vi "NMR_Long_RF_Pulse_Sequence_V4.vi"() -> ()   [LabVIEW 2020]
uses:
  <instrlib>/niFgen/niFgen.llb/niFgen Output Mode.ctl
  <instrlib>/niFgen/niFgen.llb/niFgen Waveform Type.ctl
  <instrlib>/niFgen/niFgen.llb/niFgen_ctl Trigger DigEdge - Edge Values (Ring).ctl
  <instrlib>/niFgen/niFgen.llb/niFgen_ctl Trigger Source Values (Ring).ctl
  <instrlib>/niFgen/niFgen.llb/niFgen Trigger Mode.ctl
  <instrlib>/niScope/Controls/niScope acquisition type.ctl
  <instrlib>/niScope/Controls/niScope trigger slope.ctl
  <instrlib>/niScope/Controls/niScope trigger source.ctl
  <vilib>/Analysis/2dsp.llb/Integral Method.ctl
  <vilib>/Analysis/8numeric.llb/1D Numeric Integration.vi
  <vilib>/Utility/file.llb/Read Delimited Spreadsheet (DBL).vi
  <instrlib>/niFgen/niFgen.llb/niFgen Create Waveform (DBL).vi
  <instrlib>/niScope/Configure/Trigger/niScope Configure Trigger Edge.vi
  <instrlib>/niFgen/niFgen.llb/niFgen Configure Digital Edge Start Trigger.vi
  <instrlib>/niScope/Acquire/Fetch/niScope Fetch Cluster.vi
  <vilib>/Waveform/WDTFileIO.llb/Export Waveform To Spreadsheet File.vi
  <vilib>/Analysis/NI_AALPro.lvlib
panel:
  out "Averaged T2 Decay":waveform(dbl)(graph)={"t0"=timestamp(0 s since 1904-01-01), "dt"=0.0025142857142857146, "Y"=array[865 elements]} caption="Waveform Graph"
  out "Pulse Echos - Current Scan":T1(graph) caption="Waveform Graph"
  in  "Write Output to File?":bool
  out "Scan Number":i32=1
  out "Signal Intensity (Integral)":dbl=0.2866310909595196 format="%0.4f"
  out "Extracted T2 Decay - Current Scan":waveform(dbl)(graph)={"t0"=timestamp(0 s since 1904-01-01), "dt"=0.0025142857142857146, "Y"=array[865 elements]} caption="Waveform Graph"
  in  "Pulse Train File":path=path "D:/Pulse Train - 4s Duration, 3170 Pulses, 1.25ms Tau.txt"
  in  "Larmor Frequency":dbl=27450000.0 caption="Frequency" format="%.4p"
  in  "Number of Scans":i32=16
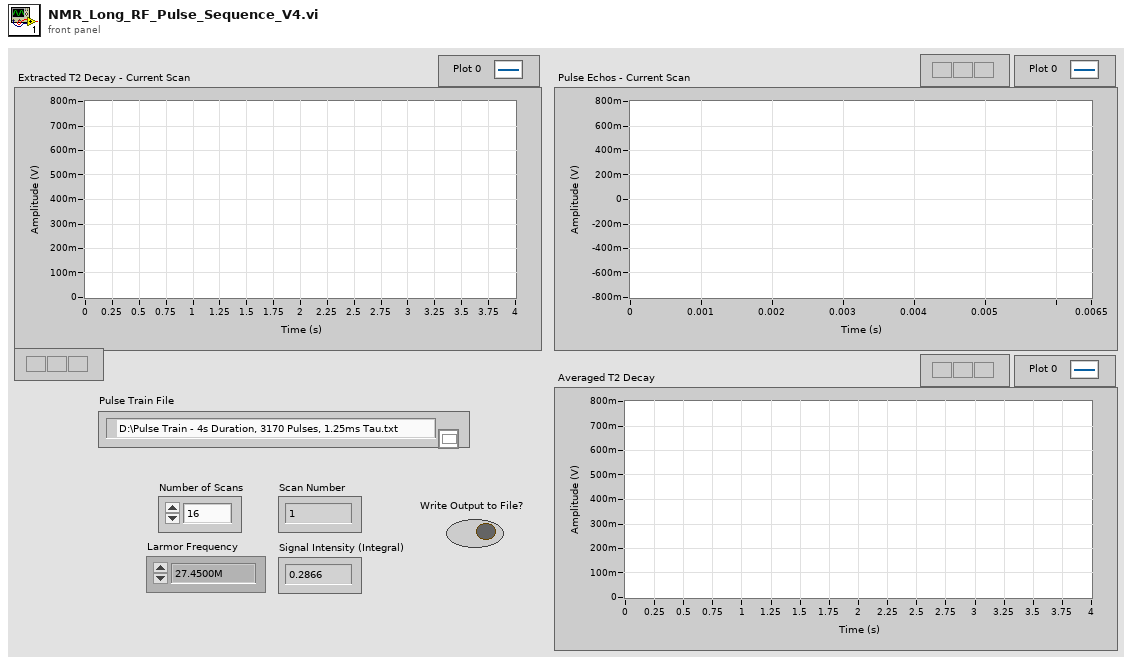
[diagram p1: front panel]
types:
  T1 = cluster{"relativeInitialX":dbl, "xIncrement":dbl, "wfm":dbl[]}
  T2 = typedef "niFgen Output Mode.ctl" = u32
  T3 = typedef "niScope trigger source.ctl" = string
  T4 = typedef "niFgen_ctl Trigger Source Values (Ring).ctl" = string
  T5 = typedef "NI_AALPro.lvlib/Integral Method.ctl" = i32
  T6 = typedef "niScope trigger slope.ctl" = i32
  T7 = typedef "niScope acquisition type.ctl" = i32
  T8 = typedef "niFgen Trigger Mode.ctl" = i32
  T9 = typedef "niFgen_ctl Trigger DigEdge - Edge Values (Ring).ctl" = i32
  T10 = typedef "niFgen Waveform Type.ctl" = i32
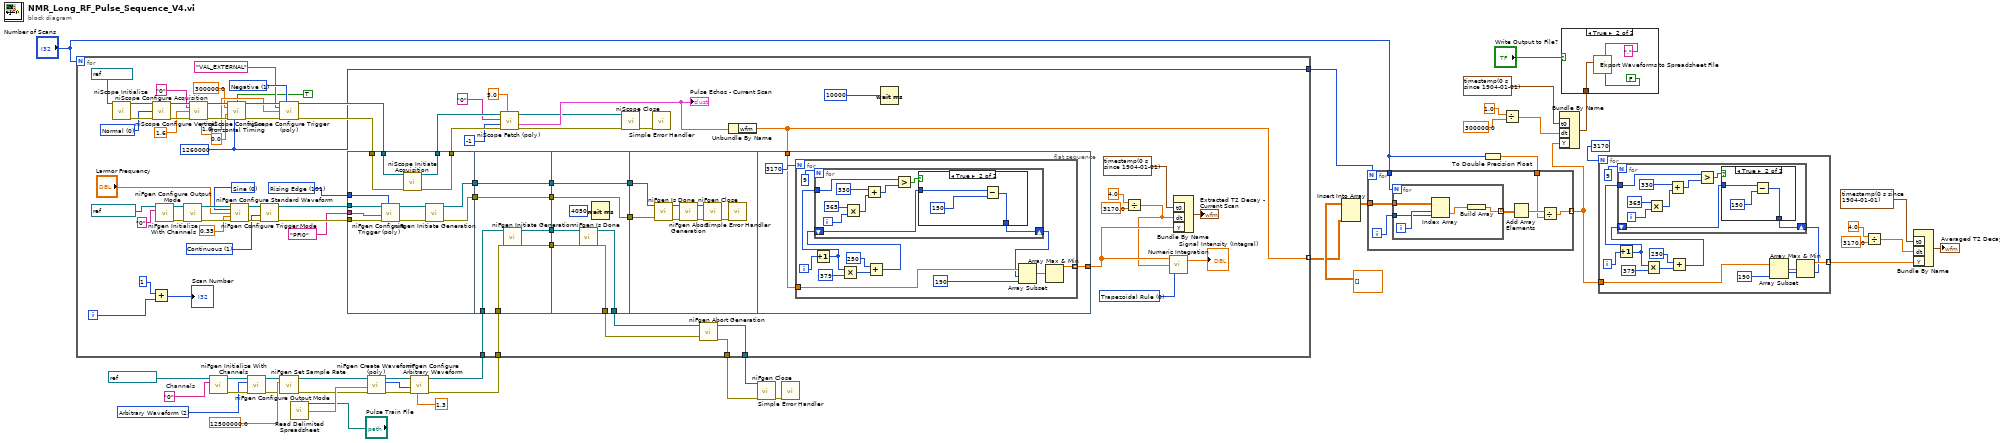
[diagram p0: block diagram]
diagram:
  w27 = "0"  # Channels
  w26 = T2 2 items=["Standard Function", "Frequency List", "Arbitrary Waveform", "Arbitrary Sequence", "Script"] ("output mode")
  n1 = call <instrlib>:"niFgen Initialize With Channels.vi"("Channel Name"=w27, "Resource Name"=refnum<k15> "PulseTrain" ("FGEN Resource Name 2")) -> ("error out"=w30:errorcluster, "Instrument Handle Out"=w31:refnum<k15>)  [unwired: 8 in]
  n2 = call <instrlib>:"niFgen Configure Output Mode.vi"("error in (no error)"=w30, "Output Mode (default: 0=Standard Function)"=w26, "Instrument Handle"=w31) -> ("error out"=w34:errorcluster, "Instrument Handle Out"=w33:refnum<k15>)  [unwired: 6 in]
  n3 = call <instrlib>:"niFgen Set Sample Rate.vi"("error in (no error)"=w34, "Sample Rate (Samp/s)"=12500000.0 ("Sample Rate"), "Instrument Handle"=w33) -> ("error out"=w37:errorcluster, "Instrument Handle Out"=w36:refnum<k15>)  [unwired: 7 in]
  n4 = call-poly <vilib>:"Read Delimited Spreadsheet.vi"("file path (dialog if empty)"="Pulse Train File") -> ("first row"=w38:dbl[])  [unwired: 9 in, 5 out]
  n5 = call-poly <instrlib>:"niFgen Create Waveform (poly).vi"("error in (no error)"=w37, "Waveform Data Array"=w38, "Instrument Handle"=w36) -> ("error out"=w40:errorcluster, "Waveform Handle"=w41:i32, "Instrument Handle Out"=w39:refnum<k15>)  [unwired: 6 in]
  n6 = call <instrlib>:"niFgen Configure Arbitrary Waveform.vi"("Gain"=1.3, "error in (no error)"=w40, "Waveform Handle"=w41, "Instrument Handle"=w39) -> ("error out"=w25:errorcluster, "Instrument Handle Out"=w24:refnum<k15>)  [unwired: 6 in]
  n7 = for {
    N: "Number of Scans" -> [_]
    tunnel: w25 -> [w96]
    tunnel: w24 -> [w95]
    tunnel: [w94] -> w22
    tunnel: [w93] -> w21
    tunnel: [w47] -> w18 mode=indexing
    tunnel: [w42] -> w9
    i -> [w50]
    w52 = T5 0 items=["Trapezoidal Rule", "Simpson's Rule", "Simpson's 3/8 Rule", "Bode Rule"] ("integration method")
    w42 = 1260000 ("min record length")
    w81 = T6 1 items=["Positive", "Negative"] ("trigger slope")
    w82 = T7 0 items=["Normal"=0, "Flex Res"=1, "DDC"=3] ("acquisition Type")
    w101 = T8 1 items=["Single", "Continuous", "Stepped", "Burst"] ("Trigger Mode (default: 1=continuous)")
    w105 = T9 101 items=["Rising Edge"=101, "Falling Edge"=102] ("Edge (Rising)")
    w106 = T10 0 items=["Sine", "Square", "Triangle", "Ramp Up", "Ramp Down", "DC", "Noise", "User"] ("Waveform")
    n8 = call <instrlib>:"niScope Initialize.vi"("resource name"=refnum<k15> "OScope") -> ("instrument handle"=w83:refnum<k15>, "error out"=w84:errorcluster)  [unwired: 13 in]
    n9 = call <instrlib>:"niScope Configure Acquisition.vi"("instrument handle"=w83, "acquisition Type"=w82, "error in"=w84) -> ("instrument handle out"=w86:refnum<k15>, "error out"=w87:errorcluster)  [unwired: 11 in]
    n10 = Add(x=1, y=w50) -> (x+y=→"Scan Number":i32)
    n11 = call <instrlib>:"niFgen Initialize With Channels.vi"("Channel Name"="0", "Resource Name"=refnum<k15> "FuncGen" ("Sine Wave Module")) -> ("error out"=w111:errorcluster, "Instrument Handle Out"=w114:refnum<k15>)  [unwired: 8 in]
    n12 = call <instrlib>:"niFgen Configure Output Mode.vi"("error in (no error)"=w111, "Instrument Handle"=w114) -> ("error out"=w110:errorcluster, "Instrument Handle Out"=w113:refnum<k15>)  [unwired: 7 in]
    n13 = call <instrlib>:"niScope Configure Vertical.vi"("instrument handle"=w86, "channels"="0", "vertical range"=1.6, "error in"=w87) -> ("instrument handle out"=w88:refnum<k15>, "error out"=w89:errorcluster)  [unwired: 10 in]
    n14 = call <instrlib>:"niScope Configure Horizontal Timing.vi"("instrument handle"=w88, "enforce realtime"=TRUE, "min sample rate"=300000.0, "reference position"=0.0, "error in"=w89, "min record length"=w42) -> ("instrument handle out"=w90:refnum<k15>, "error out"=w91:errorcluster)  [unwired: 8 in]
    n15 = call <instrlib>:"niFgen Configure Standard Waveform.vi"("Instrument Handle"=w113, "Waveform"=w106, "Frequency"="Larmor Frequency", "Amplitude"=0.35, "error in (no error)"=w110) -> ("Instrument Handle Out"=w112:refnum<k15>, "error out"=w109:errorcluster)  [unwired: 9 in]
    n16 = call <instrlib>:"niFgen Configure Trigger Mode.vi"("error in (no error)"=w109, "Trigger Mode (default: 1=continuous)"=w101, "Instrument Handle"=w112) -> ("error out"=w104:errorcluster, "Instrument Handle Out"=w102:refnum<k15>)  [unwired: 7 in]
    n17 = call-poly <instrlib>:"niScope Configure Trigger (poly).vi"("instrument handle"=w90, "trigger slope"=w81, "trigger source"=T3 "VAL_EXTERNAL", "trigger level"=1.0, "error in"=w91) -> ("instrument handle out"=w75:refnum<k15>, "error out"=w74:errorcluster)  [unwired: 9 in]
    n18 = flat-sequence {
      tunnel: w105 -> [w125]
      tunnel: w104 -> [w124]
      tunnel: T4 "PFI0" ("Source") -> [w123]
      tunnel: w102 -> [w122]
      tunnel: w75 -> [w120]
      tunnel: w74 -> [w119]
      tunnel: [w118] -> w73
      tunnel: [w117] -> w72
      tunnel: [w116] -> w62
      tunnel: [w115] -> w59
      tunnel: w96 -> [w132]
      tunnel: w95 -> [w131]
      tunnel: [w130] -> w66
      tunnel: [w129] -> w65
      tunnel: [w128] -> w63
      tunnel: w62 -> [w128]
      tunnel: [w127] -> w60
      tunnel: w59 -> [w127]
      tunnel: [w138] -> w99
      tunnel: [w137] -> w98
      tunnel: w66 -> [w136]
      tunnel: w65 -> [w135]
      tunnel: [w134] -> w64
      tunnel: w63 -> [w134]
      tunnel: [w133] -> w61
      tunnel: w60 -> [w133]
      tunnel: w64 -> [w141]
      tunnel: w61 -> [w140]
      tunnel: w47 -> [w148]
      tunnel: [w147] -> w54
      frame #0 {
        n19 = call-poly <instrlib>:"niFgen Configure Trigger (poly).vi"("Edge (Rising)"=w125, "error in (no error)"=w124, "Source"=w123, "Instrument Handle"=w122) -> ("error out"=w121:errorcluster, "Instrument Handle Out"=w126:refnum<k15>)  [unwired: 6 in]
        n20 = call <instrlib>:"niScope Initiate Acquisition.vi"("instrument handle"=w120, "error in"=w119) -> ("instrument handle out"=w118:refnum<k15>, "error out"=w117:errorcluster)  [unwired: 12 in]
        n21 = call <instrlib>:"niFgen Initiate Generation.vi"("error in (no error)"=w121, "Instrument Handle"=w126) -> ("error out"=w115:errorcluster, "Instrument Handle Out"=w116:refnum<k15>)  [unwired: 8 in]
      }
      frame #1 {
        n22 = call <instrlib>:"niFgen Initiate Generation.vi"("error in (no error)"=w132, "Instrument Handle"=w131) -> ("error out"=w129:errorcluster, "Instrument Handle Out"=w130:refnum<k15>)  [unwired: 8 in]
      }
      frame #2 {
        n23 = call <instrlib>:"niFgen Is Done.vi"("error in (no error)"=w135, "Instrument Handle"=w136) -> ("error out"=w138:errorcluster, "Instrument Handle Out"=w137:refnum<k15>)  [unwired: 7 in, 1 out]
        n24 = Wait (ms)(milliseconds to wait=u32 4050) -> ()  [unwired: 1 out]
      }
      frame #3 {
        n25 = call <instrlib>:"niFgen Is Done.vi"("error in (no error)"=w140, "Instrument Handle"=w141) -> ("error out"=w144:errorcluster, "Instrument Handle Out"=w143:refnum<k15>)  [unwired: 7 in, 1 out]
        n26 = call <instrlib>:"niFgen Abort Generation.vi"("error in (no error)"=w144, "Instrument Handle"=w143) -> ("error out"=w145:errorcluster, "Instrument Handle Out"=w146:refnum<k15>)  [unwired: 8 in]
        n27 = call <instrlib>:"niFgen Close.vi"("error in (no error)"=w145, "Instrument Handle"=w146) -> ("error out"=w142:errorcluster)  [unwired: 9 in]
        n28 = call <vilib>:"Simple Error Handler.vi"("error in (no error)"=w142) -> ()  [unwired: 4 in, 5 out]
      }
      frame #4 {
        n29 = for {
          N: 3170 -> [_]
          tunnel: [w159] -> w147 mode=indexing
          tunnel: w148 -> [w158]
          i -> [w151]
          n30 = Increment(x=w151) -> (x+1=w150:i32)
          n31 = Multiply(x=w150, y=379) -> (x*y=w157:i32)
          n32 = Add(x=250, y=w157) -> (x+y=w153:i32)
          n33 = for {
            N: 9 -> [_]
            tunnel: w150 -> [w170]
            shift-right: [w163] -> w152
            shift-left: w153 -> [w164]
            i -> [w162]
            n34 = Multiply(x=365, y=w162) -> (x*y=w166:i32)
            n35 = Add(x=330, y=w166) -> (x+y=w168:i32)
            n36 = Greater?(x=w170, y=w168) -> (0:w165:bool)
            n37 = case shown="True" w165 {
              tunnel: w164 -> [w171 w174]
              tunnel: [w171 w173] -> w163
              frame False {
              }
              frame True {
                n38 = Subtract(x=w174, y=150) -> (x-y=w173:i32)
              }
            }
          }
          n39 = Array Subset(array=w158, index=w152, length=190 ("y")) -> (w160:dbl[])
          n40 = Array Max & Min(array=w160) -> (max value=w159:dbl)  [unwired: 3 out]
        }
      }
    }
    n41 = call-poly <instrlib>:"niScope Fetch (poly).vi"("timeout"=5.0, "error in"=w72, "numSamples"=-1, "channels"="0", "instrument handle"=w73) -> ("error out"=w43:errorcluster, "waveform"=w46:T1, "instrument handle out"=w44:refnum<k15>)  [unwired: 3 in, 1 out]
    "Pulse Echos - Current Scan" <- w46
    n42 = call <instrlib>:"niScope Close.vi"("instrument handle"=w44, "error in"=w43) -> ("error out"=w92:errorcluster)  [unwired: 13 in]
    n43 = call <vilib>:"Simple Error Handler.vi"("error in (no error)"=w92) -> ()  [unwired: 4 in, 5 out]
    n44 = call <instrlib>:"niFgen Abort Generation.vi"("error in (no error)"=w99, "Instrument Handle"=w98) -> ("error out"=w94:errorcluster, "Instrument Handle Out"=w93:refnum<k15>)  [unwired: 8 in]
    n45 = Unbundle By Name(w46) -> ("wfm"=w47:dbl[])
    n46 = Wait (ms)(milliseconds to wait=u32 10000 ("Delay Time (ms)")) -> ()  [unwired: 1 out]
    n47 = Divide(x=4.0, y=3170.0) -> (x/y=w53:dbl)
    n48 = call-poly <vilib>:"Numeric Integration.vi"("integration method"=w52, "dt"=w53, "Input Array"=w54) -> ("result"=→"Signal Intensity (Integral)":dbl)  [unwired: 1 out]
    n49 = Bundle By Name("t0"=timestamp(0 s since 1904-01-01), "dt"=w53, "Y"=w54) -> (→"Extracted T2 Decay - Current Scan":waveform(dbl))  [unwired: 1 in]
  }
  n50 = call <instrlib>:"niFgen Close.vi"("error in (no error)"=w22, "Instrument Handle"=w21) -> ("error out"=w23:errorcluster)  [unwired: 9 in]
  n51 = call <vilib>:"Simple Error Handler.vi"("error in (no error)"=w23) -> ()  [unwired: 4 in, 5 out]
  n52 = Insert Into Array(array=dbl[][] [], new element=w18) -> (w20:dbl[][])  [unwired: 2 in]
  n53 = To Double Precision Float(number="Number of Scans") -> (double precision float=w17:dbl)
  n54 = for {
    N: w9 -> [_]
    tunnel: w20 -> [w181]
    tunnel: [w177] -> w2 mode=indexing
    tunnel: "Number of Scans" -> [w176]
    tunnel: w17 -> [w175]
    i -> [w180]
    n55 = for {
      N: w176 -> [_]
      tunnel: w181 -> [w186]
      tunnel: w180 -> [w184]
      tunnel: [w182] -> w179 mode=indexing
      i -> [w185]
      n56 = Index Array(array=w186, index (row)=w185, index (col)=w184) -> (element=w183:dbl)
      n57 = Build Array(w183) -> (w182:dbl[])
    }
    n58 = Add Array Elements(numeric array=w179) -> (sum=w178:dbl)
    n59 = Divide(x=w178, y=w175) -> (x/y=w177:dbl)
  }
  n60 = Divide(x=1.0, y=300000.0) -> (x/y=w12:dbl)
  n61 = Bundle By Name("t0"=timestamp(0 s since 1904-01-01), "dt"=w12, "Y"=w2) -> (w11:waveform(dbl))  [unwired: 1 in]
  n62 = case shown="True" "Write Output to File?" {
    tunnel: w11 -> [_ w187]
    frame False {
    }
    frame True {
      n63 = call-poly <vilib>:"Export Waveforms to Spreadsheet File.vi"("header? (write header:T)"=FALSE, "delimiter (Tab)"=",", "waveform"=w187) -> ()  [unwired: 7 in, 2 out]
    }
  }
  n64 = for {
    N: 3170 -> [_]
    tunnel: [w199] -> w1 mode=indexing
    tunnel: w2 -> [w198]
    i -> [w191]
    n65 = Increment(x=w191) -> (x+1=w190:i32)
    n66 = Multiply(x=w190, y=379) -> (x*y=w197:i32)
    n67 = Add(x=250, y=w197) -> (x+y=w193:i32)
    n68 = for {
      N: 9 -> [_]
      tunnel: w190 -> [w210]
      shift-right: [w203] -> w192
      shift-left: w193 -> [w204]
      i -> [w202]
      n69 = Multiply(x=365, y=w202) -> (x*y=w206:i32)
      n70 = Add(x=330, y=w206) -> (x+y=w208:i32)
      n71 = Greater?(x=w210, y=w208) -> (0:w205:bool)
      n72 = case shown="True" w205 {
        tunnel: w204 -> [w211 w214]
        tunnel: [w211 w213] -> w203
        frame False {
        }
        frame True {
          n73 = Subtract(x=w214, y=150) -> (x-y=w213:i32)
        }
      }
    }
    n74 = Array Subset(array=w198, index=w192, length=190 ("y")) -> (w200:dbl[])
    n75 = Array Max & Min(array=w200) -> (max value=w199:dbl)  [unwired: 3 out]
  }
  n76 = Divide(x=4.0, y=3170.0) -> (x/y=w4:dbl)
  n77 = Bundle By Name("t0"=timestamp(0 s since 1904-01-01), "dt"=w4, "Y"=w1) -> (→"Averaged T2 Decay":waveform(dbl))  [unwired: 1 in]
